vi "swmm_get_running.vi"(3 "error in":errorcluster, 4 "Unit system":i32(ring) items=["US", "SI"], 5 "Attribute":i32(ring) items=["Capacity"=-200, "Depth"=200, "Max. Area"=209, "Volume"=201, "Flow"=202, "Setting"=203, "Froude"=204, "Inflow"=205, "Flooding"=206, "Precipitation"=207, "Runoff"=208], 6 "object_id":string) -> (0 "error out":errorcluster, 2 "value":dbl)   [LabVIEW 2014]
uses:
  swmm5.dll
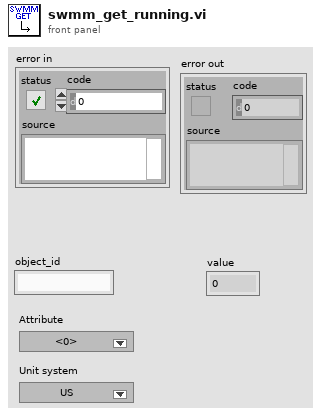
[diagram p1: front panel]
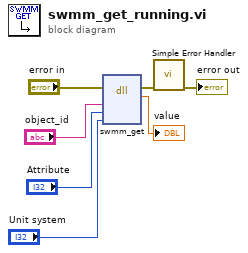
[diagram p0: block diagram]
diagram:
  n1 = dll-call lib="PTH2zabs CUsers\nandres riañoDropboxProyecto AguasSoftwareMatSWMMMatSWMM 5.1.009LabVIEW modulex64\tswmm5.dll" fn="swmm_get"(error in="error in", "object_id"="object_id", "attribute"="Attribute", "unit_system"="Unit system") -> (error out=w3:errorcluster, "return type"=→"value":dbl)  [unwired: 5 in, 1 out]
  n2 = call <vilib>:"Simple Error Handler.vi"("error in (no error)"=w3) -> ("error out"=→"error out":errorcluster)  [unwired: 4 in, 4 out]
